vi "Periodic Tasks.vi"(8 "error in":errorcluster) -> ()   [LabVIEW 2018]
doc: "This VI runs in parallel to other tasks. It can contain as many user-defined periodic loops as you need. These can carry out PID or other sorts of timed response."
uses:
  Robot Global Data.vi
panel:
  out "HAB 3:\nDrive Module Forward":bool
  out "Collector Angle Down/Out":bool
  out "Collector Angle Up/In":bool
  out "HAB 3:\nFront Cylinders Only":bool
  out "HAB 3:\nAll Cylinders":bool
  out "HAB 3:\nOverride Switches":bool
  out "HAB 3:\nBack Cylinders Only":bool
  out "Collector Angle:\nVertical":bool
  out "Collector Angle:\nDustpan Hover":bool
  out "Kick Hatch":bool
  out "Hatch Retainer\nUp/Down":bool
  out "wrong answer":bool
  out "SCORE":dbl
  out "STEAK":dbl
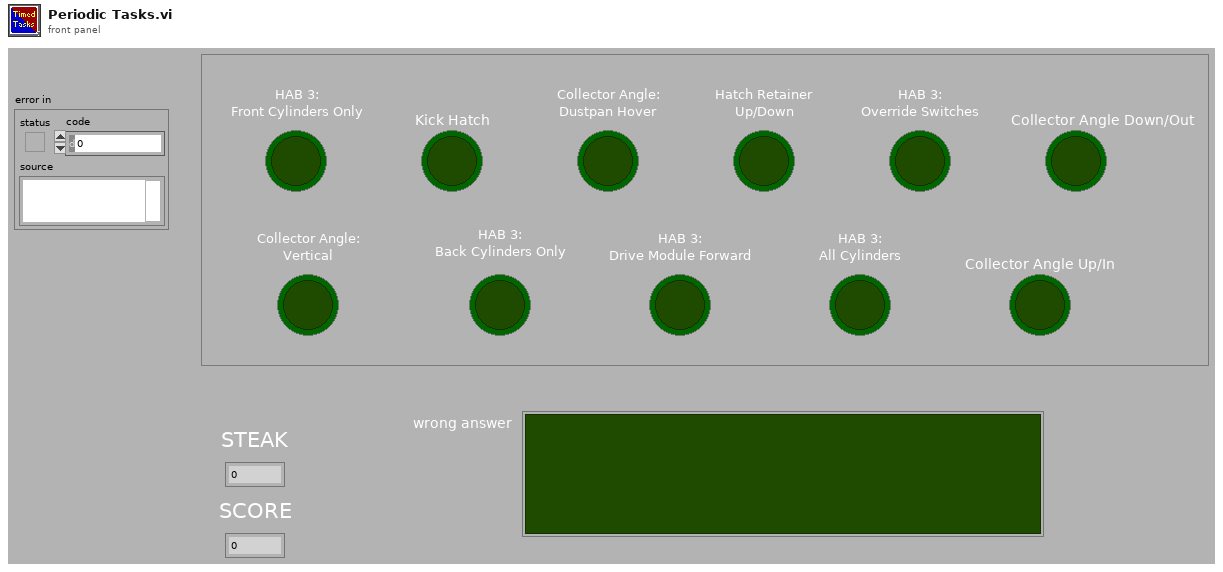
[diagram p1: front panel]
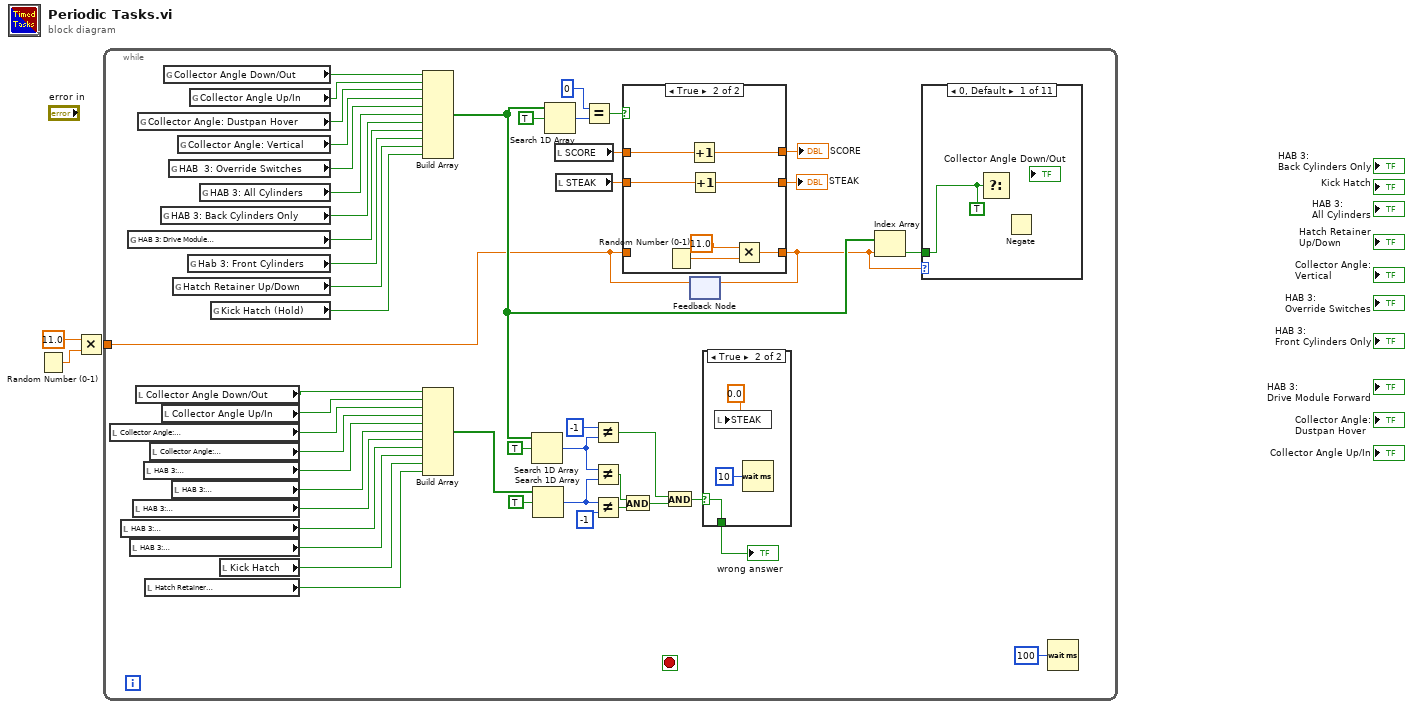
[diagram p0: block diagram]
diagram:
  n1 = Random Number (0-1)() -> (number: 0 to 1=w2:dbl)
  n2 = Multiply(x=11.0, y=w2) -> ()  [unwired: 1 out]
  n3 = while {
    tunnel: [w4] -> _
    stop <- _ stop-if-true
    n4 = local read "Collector Angle:\nDustpan Hover"() -> (w13:bool)
    n5 = local read "HAB 3:\nDrive Module Forward"() -> (w8:bool)
    n6 = global read "Robot Global Data.vi" "HAB 3: Drive Module\n(FORWARD)"() -> (w43:bool)
    n7 = local read "HAB 3:\nFront Cylinders Only"() -> (w7:bool)
    n8 = local read "HAB 3:\nBack Cylinders Only"() -> (w9:bool)
    n9 = local read "Collector Angle Down/Out"() -> (w15:bool)
    n10 = global read "Robot Global Data.vi" "Collector Angle: Dustpan Hover"() -> (w48:bool)
    n11 = local read "HAB 3:\nOverride Switches"() -> (w11:bool)
    n12 = local read "Hatch Retainer\nUp/Down"() -> (w5:bool)
    n13 = local read "Collector Angle:\nVertical"() -> (w12:bool)
    n14 = global read "Robot Global Data.vi" "HAB 3: Back Cylinders Only"() -> (w44:bool)
    n15 = local read "Collector Angle Up/In"() -> (w14:bool)
    n16 = global read "Robot Global Data.vi" "Collector Angle Down/Out"() -> (w50:bool)
    n17 = global read "Robot Global Data.vi" "HAB  3: Override Switches"() -> (w46:bool)
    n18 = local read "HAB 3:\nAll Cylinders"() -> (w10:bool)
    n19 = global read "Robot Global Data.vi" "Hatch Retainer Up/Down"() -> (w41:bool)
    n20 = global read "Robot Global Data.vi" "Collector Angle: Vertical"() -> (w47:bool)
    n21 = global read "Robot Global Data.vi" "Hab 3: Front Cylinders"() -> (w42:bool)
    n22 = global read "Robot Global Data.vi" "Collector Angle Up/In"() -> (w49:bool)
    n23 = global read "Robot Global Data.vi" "HAB 3: All Cylinders"() -> (w45:bool)
    n24 = global read "Robot Global Data.vi" "Kick Hatch (Hold)"() -> (w40:bool)
    n25 = local read "Kick Hatch"() -> (w6:bool)
    n26 = Build Array(w50, w49, w48, w47, w46, w45, w44, w43, w42, w41, w40) -> (w17:bool[])
    n27 = Build Array(w15, w14, w13, w12, w11, w10, w9, w8, w7, w6, w5) -> (w18:bool[])
    n28 = Search 1D Array(1D array=w17, element=TRUE) -> (index of element=w22:i32)  [unwired: 1 in]
    n29 = Search 1D Array(1D array=w18, element=TRUE) -> (index of element=w25:i32)  [unwired: 1 in]
    n30 = Search 1D Array(1D array=w17, element=TRUE) -> (index of element=w38:i32)  [unwired: 1 in]
    n31 = local read "SCORE"() -> (w35:dbl)
    n32 = local read "STEAK"() -> (w32:dbl)
    n33 = Equal?(x=0, y=w38) -> (x = y?=w36:bool)
    n34 = Not Equal?(x=-1, y=w22) -> (x != y?=w20:bool)
    n35 = Not Equal?(x=w22, y=w25) -> (x != y?=w27:bool)
    n36 = Not Equal?(x=w25, y=-1 ("x")) -> (x != y?=w28:bool)
    n37 = And(x=w27, y=w28) -> (x .and. y?=w23:bool)
    n38 = And(x=w20, y=w23) -> (x .and. y?=w29:bool)
    n39 = feedback #1() -> (w4:dbl)  [unwired: 1 in]
    n40 = case shown="True" w36 {
      tunnel: w35 -> [w58 w65]
      tunnel: [w58 w64] -> w34
      tunnel: [w57 w62] -> w33
      tunnel: w32 -> [w57 w63]
      tunnel: w4 -> [w56 _]
      tunnel: [w56 w59] -> w16
      frame False {
      }
      frame True {
        n41 = Random Number (0-1)() -> (number: 0 to 1=w61:dbl)
        n42 = Increment(x=w65) -> (x+1=w64:dbl)
        n43 = Increment(x=w63) -> (x+1=w62:dbl)
        n44 = Multiply(x=11.0, y=w61) -> (x*y=w59:dbl)
      }
    }
    "STEAK" <- w33
    "SCORE" <- w34
    n45 = feedback-in #1(w16) -> ()
    n46 = case shown="True" w29 {
      selector: w29 -> [w51 w52]
      tunnel: [w51 w52] -> w19
      frame False {
      }
      frame True {
        n47 = local write "STEAK"(0.0) -> ()
        n48 = Wait (ms)(milliseconds to wait=u32 10) -> ()  [unwired: 1 out]
      }
    }
    "wrong answer" <- w19
    n49 = Index Array(array=w17, index=w16) -> (element=w3:bool)
    n50 = case shown="0, Default" w16 {
      tunnel: [w55 _ _ _ _ _ _ _ _ _ _] -> _
      tunnel: w3 -> [_ _ _ _ _ _ _ _ _ _ _]
      frame 0, Default {
        w55 = TRUE
        n51 = Select(s=w55) -> ()  [unwired: 2 in, 1 out]
        n52 = Negate() -> ()  [unwired: 1 in, 1 out]
      }
      frame 3 {
      }
      frame 4 {
      }
      frame 5 {
      }
      frame 6 {
      }
      frame 7 {
      }
      frame 8 {
      }
      frame 9 {
      }
      frame 10 {
      }
      frame 1 {
      }
      frame 2 {
      }
    }
    n53 = Wait (ms)(milliseconds to wait=u32 100) -> ()  [unwired: 1 out]
  }
